vi "GEA2 FP ERD Parse.vi"(8 "Error In":errorcluster, 10 "Header":string[](array[string]), 11 "ERD Data Out":T1[](array[typedef]) {"ERD Number" format="%.0x"}) -> (0 "Error Out":errorcluster, 3 "Array out":string[][](array[string]))   [LabVIEW 2016]
uses:
  type defs/ERD Read Data Out.ctl
  library/GEA2_Toolkit.lvlib
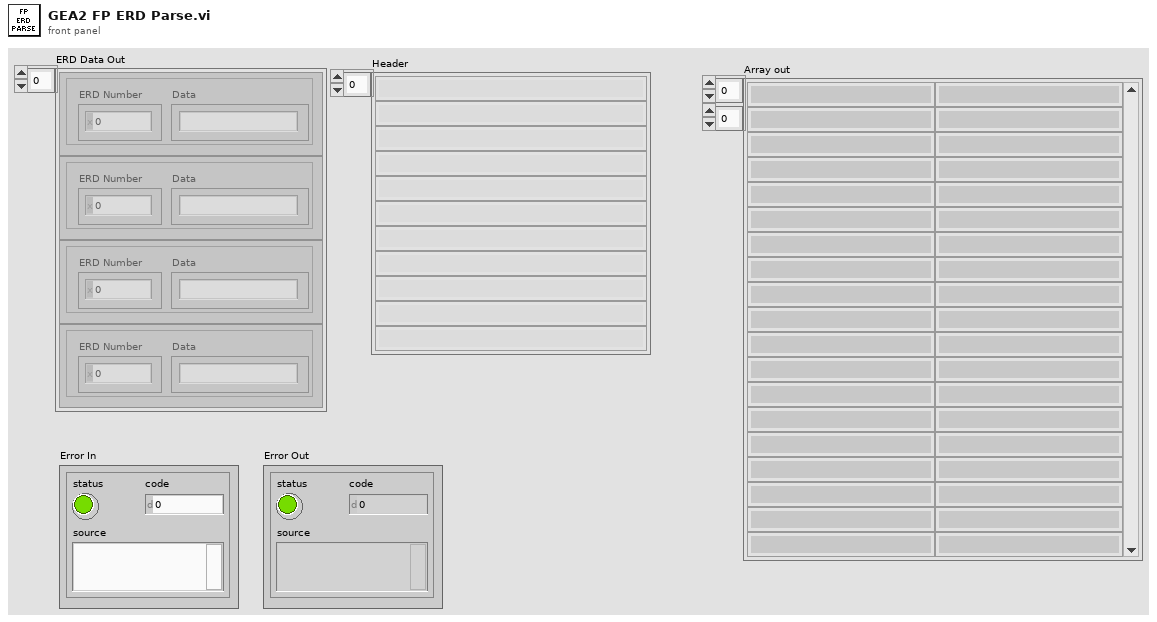
[diagram p1: front panel]
types:
  T1 = typedef "GEA2_Toolkit.lvlib/ERD Read Data Out.ctl" = cluster{"ERD Number":u16, "Data":string}
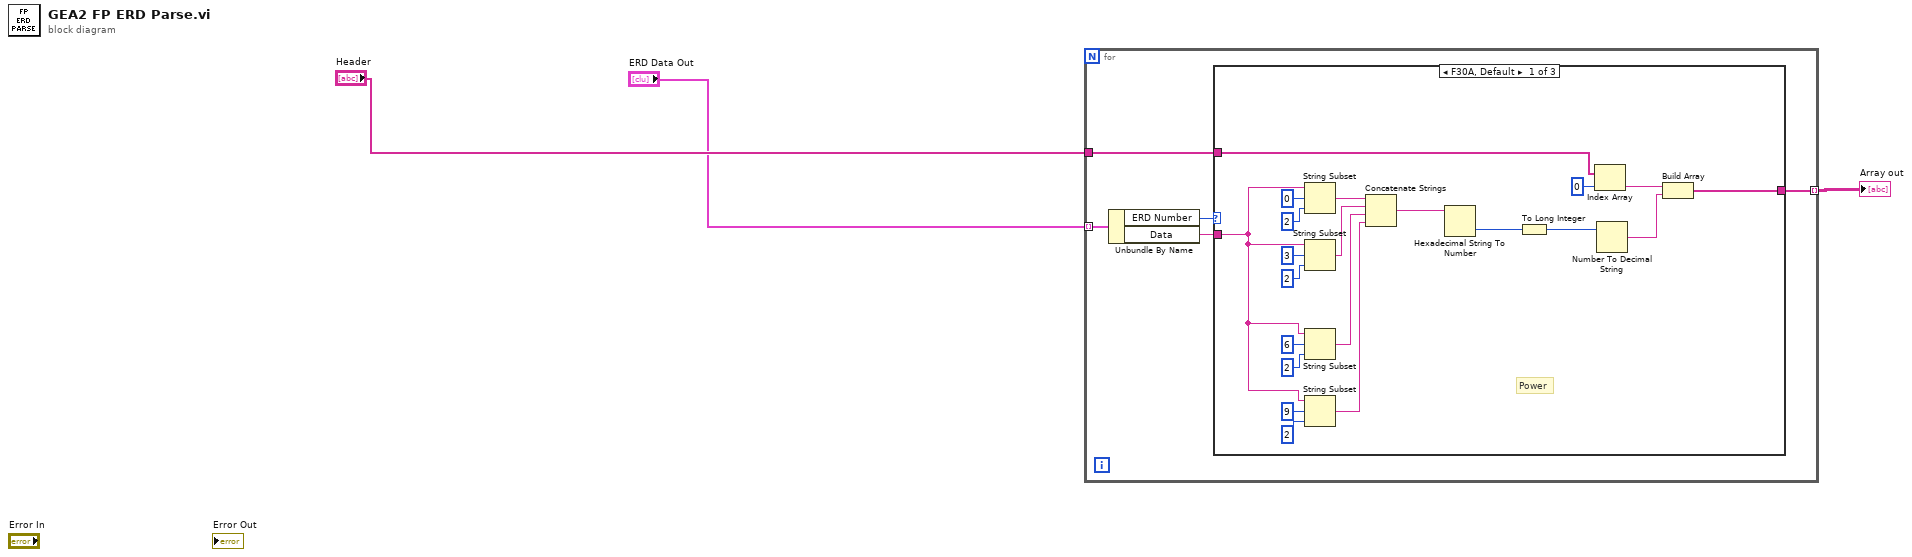
[diagram p0: block diagram]
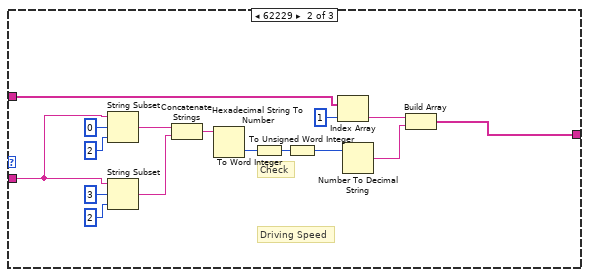
[diagram p2: hidden frame]
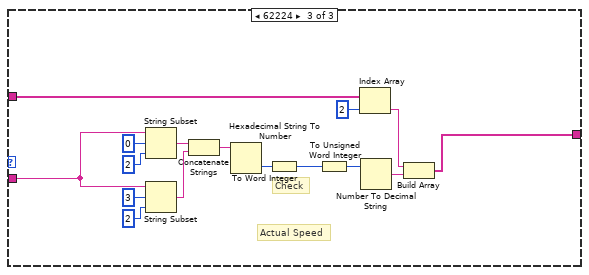
[diagram p3: hidden frame]
diagram:
  n1 = for {
    tunnel: "ERD Data Out" -> [w8] mode=indexing
    tunnel: "Header" -> [w6]
    tunnel: [w4] -> w3 mode=indexing
    n2 = Unbundle By Name(w8) -> ("ERD Number"=w7:u16, "Data"=w5:string)
    n3 = case shown="F30A, Default" w7 {
      tunnel: w6 -> [w11 w32 w48]
      tunnel: w5 -> [w10 w31 w47]
      tunnel: [w9 w30 w46] -> w4
      frame 62218, Default {
        # "Power"
        n4 = String Subset(string=w10, offset (0)=0, length (rest)=2 ("length (rest)")) -> (substring=w25:string)
        n5 = String Subset(string=w10, offset (0)=3, length (rest)=2 ("length (rest)")) -> (substring=w24:string)
        n6 = String Subset(string=w10, offset (0)=6, length (rest)=2 ("length (rest)")) -> (substring=w17:string)
        n7 = String Subset(string=w10, offset (0)=9, length (rest)=2 ("length (rest)")) -> (substring=w16:string)
        n8 = Concatenate Strings(w25, w24, w17, w16) -> (w23:string)
        n9 = Hexadecimal String To Number(string=w23) -> (number=w22:u32)  [unwired: 2 in, 1 out]
        n10 = To Long Integer(number=w22) -> (32bit integer=w15:i32)
        n11 = Index Array(array=w11, index=0) -> (element=w13:string)
        n12 = Number To Decimal String(number=w15) -> (decimal integer string=w12:string)  [unwired: 1 in]
        n13 = Build Array(w13, w12) -> (w9:string[])
      }
      frame 62229 {
        # "Driving Speed"
        # "Check"
        n14 = String Subset(string=w31, offset (0)=0, length (rest)=2 ("length (rest)")) -> (substring=w39:string)
        n15 = String Subset(string=w31, offset (0)=3, length (rest)=2 ("length (rest)")) -> (substring=w38:string)
        n16 = Concatenate Strings(w39, w38) -> (w37:string)
        n17 = Hexadecimal String To Number(string=w37) -> (number=w36:u32)  [unwired: 2 in, 1 out]
        n18 = To Word Integer(number=w36) -> (16bit integer=w33:i16)
        n19 = To Unsigned Word Integer(number=w33) -> (unsigned 16bit integer=w35:u16)
        n20 = Index Array(array=w32, index=1) -> (element=w44:string)
        n21 = Number To Decimal String(number=w35) -> (decimal integer string=w34:string)  [unwired: 1 in]
        n22 = Build Array(w44, w34) -> (w30:string[])
      }
      frame 62224 {
        # "Actual Speed"
        # "Check"
        n23 = String Subset(string=w47, offset (0)=0, length (rest)=2 ("length (rest)")) -> (substring=w55:string)
        n24 = String Subset(string=w47, offset (0)=3, length (rest)=2 ("length (rest)")) -> (substring=w56:string)
        n25 = Concatenate Strings(w55, w56) -> (w57:string)
        n26 = Hexadecimal String To Number(string=w57) -> (number=w58:u32)  [unwired: 2 in, 1 out]
        n27 = To Word Integer(number=w58) -> (16bit integer=w61:i16)
        n28 = To Unsigned Word Integer(number=w61) -> (unsigned 16bit integer=w59:u16)
        n29 = Index Array(array=w48, index=2) -> (element=w50:string)
        n30 = Number To Decimal String(number=w59) -> (decimal integer string=w60:string)  [unwired: 1 in]
        n31 = Build Array(w50, w60) -> (w46:string[])
      }
    }
  }
  "Array out" <- w3
